vi "PhotoDetSyringeZ.vi"(0 "GoToPhotoDetector":string="G90\nG1 Z0 F100\nG1 X1107.333\tY32.555\nG1\tZ80 F50\nG1\tZ86 F1", 11 "Error In":errorcluster) -> (2 "Vmax":dbl, 3 "Vstart":dbl, 4 "Zfinal":dbl, 10 "VatZfinal":dbl, 13 "Vmin":dbl, 14 "Vmid":dbl, 15 "error out":errorcluster)   [LabVIEW 2019]
panel:
  out "VmidViDiff":dbl[](array[numeric])
  out "ZmidScan":dbl[](array[numeric])
  out "VmidScan":dbl[](array[numeric])
  out "ZstopVminScan":dbl
  out "ZstopVmaxScan":dbl
  out "XYZinLimits":bool
  in  "ZupLim":dbl=89.0 format="%#_7g"
  in  "ZlowLim":dbl=85.0 format="%#_7g"
  in  "YupLim":dbl=32.8 format="%#_7g"
  in  "YlowLim":dbl=32.2 format="%#_7g"
  in  "XupLim":dbl=1107.5 format="%#_7g"
  in  "XlowLim":dbl=1107.0 format="%#_7g"
  in  "Status":string
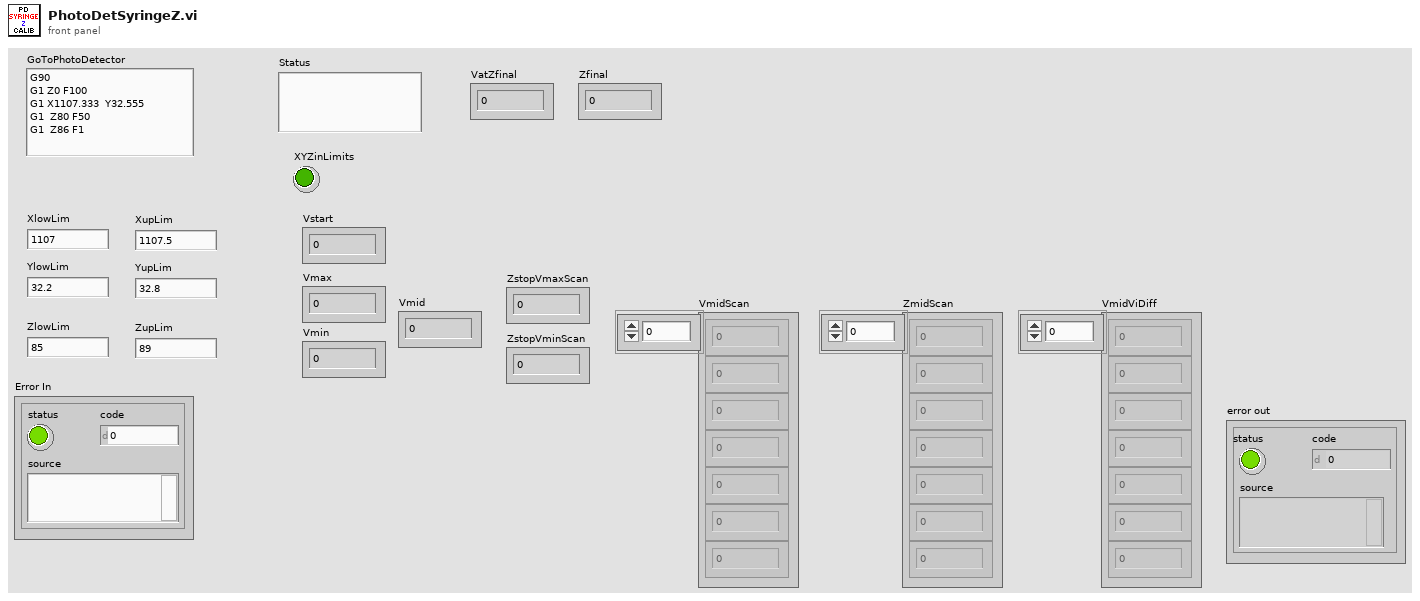
[diagram p1: front panel]
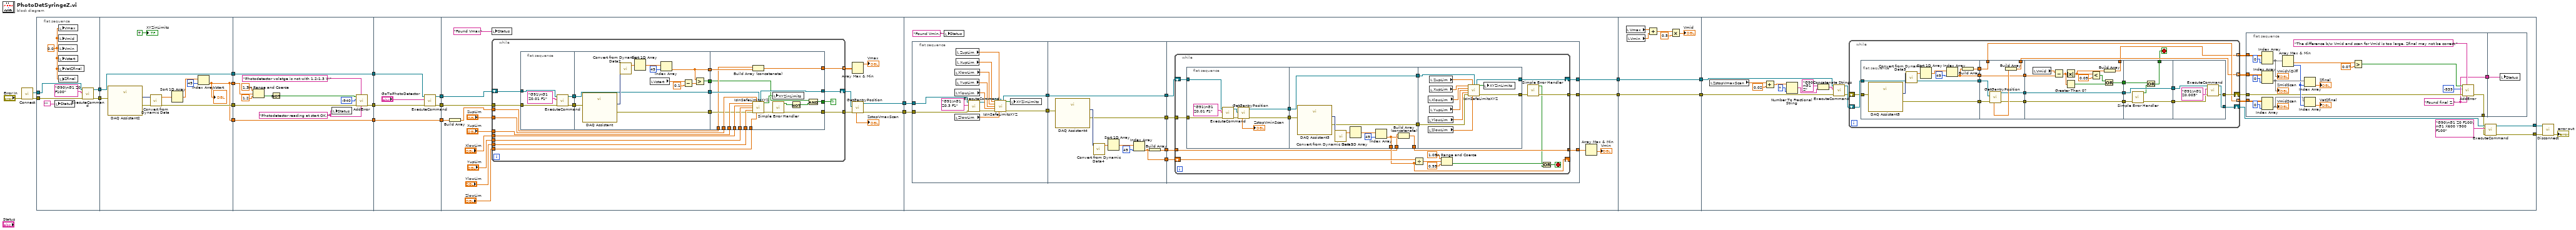
[diagram p0: block diagram]
diagram:
  n1 = call "Connect.vi"("error in (no error)"="Error In") -> ("error out"=w2:errorcluster, "controller"=w1:refnum<k24>)  [unwired: 9 in]
  n2 = flat-sequence {
    tunnel: [w30] -> w24
    tunnel: [w29] -> w19
    tunnel: w2 -> [w27]
    tunnel: w1 -> [w26]
    tunnel: w24 -> [w36]
    tunnel: [w35] -> w23
    tunnel: [w32] -> w22
    tunnel: [w34] -> w20
    tunnel: w19 -> [w34]
    tunnel: [w32] -> w15
    tunnel: w23 -> [w52]
    tunnel: w22 -> [w49]
    tunnel: [w44] -> w21
    tunnel: w20 -> [w44]
    tunnel: [w43] -> w18
    tunnel: w15 -> [w41]
    tunnel: [w41] -> w13
    tunnel: w21 -> [w57]
    tunnel: w18 -> [w56]
    tunnel: [w55] -> w17
    tunnel: [w54] -> w16
    tunnel: [w53] -> w14
    tunnel: w13 -> [w53]
    tunnel: w17 -> [w71]
    tunnel: w16 -> [w76]
    tunnel: w14 -> [w75]
    tunnel: [w61] -> w12
    tunnel: [w60] -> w11
    tunnel: w12 -> [w143]
    tunnel: w11 -> [w144]
    tunnel: [w137] -> w9
    tunnel: [w136] -> w8
    tunnel: w9 -> [w229]
    tunnel: w8 -> [w228]
    tunnel: [w229] -> w7
    tunnel: [w228] -> w6
    tunnel: w7 -> [w247]
    tunnel: w6 -> [w246]
    tunnel: [w231] -> w5
    tunnel: [w234] -> w4
    frame #0 {
      w25 = 0.0 ("Vmax")
      n3 = local write "Status"("") -> ()
      n4 = local write "Vmax"(w25) -> ()
      n5 = local write "Vmid"(w25) -> ()
      n6 = local write "Vmin"(w25) -> ()
      n7 = local write "Vstart"(w25) -> ()
      n8 = local write "VatZfinal"(w25) -> ()
      n9 = local write "Zfinal"(w25) -> ()
      n10 = call "ExecuteCommand.vi"("error in (no error)"=w27, "Command Code"="G90\nG1 Z0 F100", "controller in"=w26) -> ("error out"=w30:errorcluster, "controller out"=w29:refnum<k24>)  [unwired: 6 in, 1 out]
    }
    frame #1 {
      n11 = call "DAQ Assistant2"("error in"=w36) -> ("data"=w40:dynamicdata, "error out"=w35:errorcluster)  [unwired: 16 in, 1 out]
      n12 = call "Convert from Dynamic Data"("Dynamic Data Type"=w40) -> ("Array"=w39:dbl[])  [unwired: 3 in]
      n13 = Sort 1D Array(array=w39) -> (sorted array=w38:dbl[])
      n14 = Index Array(array=w38, index=49) -> (element=w32:dbl)
      "Vstart" <- w32
      "XYZinLimits" <- TRUE ("XYZinLimits")
    }
    frame #2 {
      w42 = "Photodetector reading at start OK." ("NoErrorMessage")
      n15 = In Range and Coerce(upper limit=1.3, x=w49, lower limit=1.2) -> (In Range?=w51:bool)  [unwired: 1 out]
      n16 = Not(x=w51) -> (.not. x?=w47:bool)
      n17 = local write "Status"(w42) -> ()
      n18 = call "AddError.vi"("NoErrorMessage"=w42, "ErrorMessage"="Photodetector volatge is not with 1.2-1.3 V.", "error in"=w52, "code"=-940, "Error?"=w47) -> ("Error out"=w43:errorcluster)  [unwired: 6 in]
    }
    frame #3 {
      n19 = call "ExecuteCommand.vi"("error in (no error)"=w56, "Command Code"="GoToPhotoDetector", "controller in"=w57) -> ("error out"=w55:errorcluster, "controller out"=w54:refnum<k24>)  [unwired: 6 in, 1 out]
    }
    frame #4 {
      n20 = Build Array(w75) -> (w74:dbl[])
      n21 = local write "Status"("Found Vmax" ("NoErrorMessage")) -> ()
      n22 = while {
        shift-right: [w82] -> w64
        shift-left: w76 -> [w95]
        tunnel: "XlowLim" -> [w94]
        tunnel: "XupLim" -> [w93]
        tunnel: "YlowLim" -> [w92]
        tunnel: "YupLim" -> [w91]
        tunnel: "ZupLim" -> [w90]
        tunnel: "ZlowLim" -> [w89]
        tunnel: w74 -> [w83]
        tunnel: [w81] -> w73 mode=indexing
        tunnel: [w80] -> w63
        tunnel: w71 -> [w79]
        stop <- w77 continue-if-true
        n23 = flat-sequence {
          tunnel: w95 -> [w99]
          tunnel: [w98] -> w88
          tunnel: [w97] -> w85
          tunnel: w79 -> [w96]
          tunnel: w88 -> [w108]
          tunnel: [w108] -> w87
          tunnel: [w102] -> w86
          tunnel: w85 -> [w107]
          tunnel: [w104] -> w84
          tunnel: [w101] -> w78
          tunnel: w94 -> [w131]
          tunnel: w93 -> [w130]
          tunnel: w92 -> [w129]
          tunnel: w91 -> [w128]
          tunnel: w90 -> [w127]
          tunnel: w89 -> [w126]
          tunnel: w87 -> [w125]
          tunnel: w86 -> [w123]
          tunnel: w84 -> [w122]
          tunnel: w83 -> [w121]
          tunnel: [w120] -> w82
          tunnel: [w119] -> w81
          tunnel: [w117] -> w80
          tunnel: w78 -> [w116]
          tunnel: [w115] -> w77
          frame #0 {
            n24 = call "ExecuteCommand.vi"("error in (no error)"=w96, "Command Code"="G91\nG1 Z0.01 F1", "controller in"=w99) -> ("error out"=w97:errorcluster, "controller out"=w98:refnum<k24>)  [unwired: 6 in, 1 out]
          }
          frame #1 {
            n25 = call "DAQ Assistant"("error in"=w107) -> ("data"=w112:dynamicdata, "error out"=w102:errorcluster)  [unwired: 16 in, 1 out]
            n26 = call "Convert from Dynamic Data2"("Dynamic Data Type"=w112) -> ("Array"=w111:dbl[])  [unwired: 3 in]
            n27 = Sort 1D Array(array=w111) -> (sorted array=w110:dbl[])
            n28 = local read "Vstart"() -> (w106:dbl)
            n29 = Index Array(array=w110, index=49) -> (element=w104:dbl)
            n30 = Subtract(x=w106, y=0.1) -> (x-y=w103:dbl)
            n31 = Greater?(x=w104, y=w103) -> (0:w101:bool)
          }
          frame #2 {
            n32 = Build Array (concatenate)(w121, w122) -> (w119:dbl[])
            n33 = call "IsInSafeLimitsXYZ.vi"("XupLim"=w130, "ZupLim"=w127, "Controller In"=w125, "XlowLim"=w131, "YupLim"=w128, "YlowLim"=w129, "Error In"=w123, "ZlowLim"=w126) -> ("controller out"=w120:refnum<k24>, "XYZinLimits"=w124:bool, "Error Out"=w118:errorcluster)  [unwired: 5 in]
            n34 = local write "XYZinLimits"(w124) -> ()
            n35 = call <vilib>:"Simple Error Handler.vi"("error in (no error)"=w118) -> ("error?"=w113:bool, "error out"=w117:errorcluster)  [unwired: 4 in, 3 out]
            n36 = Not(x=w113) -> (.not. x?=w114:bool)
            n37 = And(x=w116, y=w114) -> (x .and. y?=w115:bool)
          }
        }
      }
      n38 = Array Max & Min(array=w73) -> (max value=→"Vmax":dbl)  [unwired: 3 out]
      n39 = call "GetGantryPosition.vi"("error in (no error)"=w63, "Controller In"=w64) -> ("error out"=w61:errorcluster, "controller out"=w60:refnum<k24>, "Position Z"=→"ZstopVmaxScan":dbl)  [unwired: 3 in, 4 out]
    }
    frame #5 {
      n40 = flat-sequence {
        tunnel: w144 -> [w158]
        tunnel: w143 -> [w156]
        tunnel: [w146] -> w142
        tunnel: [w147] -> w139
        tunnel: w142 -> [w163]
        tunnel: [w162] -> w141
        tunnel: [w160] -> w140
        tunnel: w139 -> [w161]
        tunnel: [w161] -> w138
        tunnel: [w159] -> w135
        tunnel: w141 -> [w174]
        tunnel: w140 -> [w173]
        tunnel: w138 -> [w172]
        tunnel: [w168] -> w137
        tunnel: [w171] -> w136
        tunnel: w135 -> [w170]
        tunnel: [w169] -> w134
        frame #0 {
          n41 = local read "XlowLim"() -> (w154:dbl)
          n42 = local read "YlowLim"() -> (w152:dbl)
          n43 = local read "ZlowLim"() -> (w150:dbl)
          n44 = local read "ZupLim"() -> (w149:dbl)
          n45 = local read "XupLim"() -> (w153:dbl)
          n46 = local read "YupLim"() -> (w151:dbl)
          n47 = call "ExecuteCommand.vi"("error in (no error)"=w156, "Command Code"="G91\nG1 Z0.3 F1", "controller in"=w158) -> ("error out"=w155:errorcluster, "controller out"=w148:refnum<k24>)  [unwired: 6 in, 1 out]
          n48 = call "IsInSafeLimitsXYZ.vi"("XupLim"=w153, "ZupLim"=w149, "Controller In"=w148, "XlowLim"=w154, "YupLim"=w151, "YlowLim"=w152, "Error In"=w155, "ZlowLim"=w150) -> ("controller out"=w147:refnum<k24>, "XYZinLimits"=w145:bool, "Error Out"=w146:errorcluster)  [unwired: 5 in]
          n49 = local write "XYZinLimits"(w145) -> ()
        }
        frame #1 {
          n50 = call "DAQ Assistant4"("error in"=w163) -> ("data"=w164:dynamicdata, "error out"=w162:errorcluster)  [unwired: 16 in, 1 out]
          n51 = call "Convert from Dynamic Data4"("Dynamic Data Type"=w164) -> ("Array"=w167:dbl[])  [unwired: 3 in]
          n52 = Sort 1D Array(array=w167) -> (sorted array=w166:dbl[])
          n53 = Index Array(array=w166, index=49) -> (element=w160:dbl)
          n54 = Build Array(w160) -> (w159:dbl[])
        }
        frame #2 {
          n55 = while {
            shift-right: [w189] -> _
            shift-left: w173 -> [w190]
            shift-right: [w183] -> w171
            shift-left: w172 -> [w191]
            tunnel: w170 -> [w181]
            tunnel: [w180] -> w169 mode=concatenating
            tunnel: w174 -> [w193]
            tunnel: [w178] -> w168
            stop <- w175 stop-if-true
            n56 = flat-sequence {
              tunnel: w193 -> [w199]
              tunnel: [w195] -> w192
              tunnel: w191 -> [w200]
              tunnel: [w197] -> w185
              tunnel: w192 -> [w207]
              tunnel: [w204] -> w189
              tunnel: w185 -> [w206]
              tunnel: [w206] -> w184
              tunnel: [w205] -> w182
              tunnel: w181 -> [w203]
              tunnel: [w202] -> w180
              tunnel: w184 -> [w215]
              tunnel: [w214] -> w183
              tunnel: w182 -> [w213]
              tunnel: [w212] -> w179
              frame #0 {
                n57 = call "ExecuteCommand.vi"("error in (no error)"=w199, "Command Code"="G91\nG1 Z0.01 F1", "controller in"=w200) -> ("error out"=w194:errorcluster, "controller out"=w198:refnum<k24>)  [unwired: 6 in, 1 out]
                n58 = call "GetGantryPosition.vi"("error in (no error)"=w194, "Controller In"=w198) -> ("error out"=w195:errorcluster, "controller out"=w197:refnum<k24>, "Position Z"=→"ZstopVminScan":dbl)  [unwired: 3 in, 4 out]
              }
              frame #1 {
                n59 = call "DAQ Assistant3"("error in"=w207) -> ("data"=w208:dynamicdata, "error out"=w205:errorcluster)  [unwired: 16 in, 1 out]
                n60 = call "Convert from Dynamic Data3"("Dynamic Data Type"=w208) -> ("Array"=w211:dbl[])  [unwired: 3 in]
                n61 = Sort 1D Array(array=w211) -> (sorted array=w210:dbl[])
                n62 = Index Array(array=w210, index=49) -> (element=w204:dbl)
                n63 = Build Array (concatenate)(w203, w204) -> (w202:dbl[])
              }
              frame #2 {
                n64 = local read "XlowLim"() -> (w222:dbl)
                n65 = local read "YlowLim"() -> (w219:dbl)
                n66 = local read "ZlowLim"() -> (w217:dbl)
                n67 = local read "ZupLim"() -> (w218:dbl)
                n68 = local read "XupLim"() -> (w221:dbl)
                n69 = local read "YupLim"() -> (w220:dbl)
                n70 = call "IsInSafeLimitsXYZ.vi"("XupLim"=w221, "ZupLim"=w218, "Controller In"=w215, "XlowLim"=w222, "YupLim"=w220, "YlowLim"=w219, "Error In"=w213, "ZlowLim"=w217) -> ("controller out"=w214:refnum<k24>, "XYZinLimits"=w216:bool, "Error Out"=w212:errorcluster)  [unwired: 5 in]
                n71 = local write "XYZinLimits"(w216) -> ()
              }
            }
            n72 = Divide(x=w190, y=w189) -> (x/y=w188:dbl)
            n73 = In Range and Coerce(upper limit=1.05, x=w188, lower limit=0.95) -> (In Range?=w177:bool)  [unwired: 1 out]
            n74 = call <vilib>:"Simple Error Handler.vi"("error in (no error)"=w179) -> ("error?"=w176:bool, "error out"=w178:errorcluster)  [unwired: 4 in, 3 out]
            n75 = Or(x=w177, y=w176) -> (x .or. y?=w175:bool)
          }
        }
      }
      n76 = local write "Status"("Found Vmin." ("Status")) -> ()
      n77 = Array Max & Min(array=w134) -> (min value=→"Vmin":dbl)  [unwired: 3 out]
    }
    frame #6 {
      n78 = local read "Vmax"() -> (w226:dbl)
      n79 = local read "Vmin"() -> (w225:dbl)
      n80 = Add(x=w226, y=w225) -> (x+y=w224:dbl)
      n81 = Multiply(x=w224, y=0.5) -> (x*y=→"Vmid":dbl)
    }
    frame #7 {
      n82 = local read "ZstopVmaxScan"() -> (w248:dbl)
      n83 = Add(x=w248, y=0.02) -> (x+y=w249:dbl)
      n84 = Number To Fractional String(number=w249, precision (6)=i16 7) -> (F-format string=w250:string)  [unwired: 2 in]
      n85 = Concatenate Strings("G90\nG1 Z", w250) -> (w242:string)
      n86 = call "ExecuteCommand.vi"("error in (no error)"=w247, "Command Code"=w242, "controller in"=w246) -> ("error out"=w240:errorcluster, "controller out"=w241:refnum<k24>)  [unwired: 6 in, 1 out]
      n87 = while {
        shift-right: [w286] -> w235
        shift-left: w241 -> [w289]
        shift-right: [w283] -> w230
        shift-left: w240 -> [w282]
        tunnel: [w281] -> w237 mode=indexing
        tunnel: [w279] -> w238 mode=indexing
        tunnel: [w272] -> w239 mode=indexing
        stop <- w273 stop-if-true
        n88 = flat-sequence {
          tunnel: w282 -> [w296]
          tunnel: [w295] -> w291
          tunnel: w289 -> [w294]
          tunnel: [w294] -> w288
          tunnel: [w293] -> w285
          tunnel: [w292] -> w280
          tunnel: w291 -> [w307]
          tunnel: [w307] -> w290
          tunnel: w288 -> [w306]
          tunnel: [w305] -> w287
          tunnel: w285 -> [w304]
          tunnel: [w303] -> w284
          tunnel: [w302] -> w281
          tunnel: w280 -> [w302]
          tunnel: [w301] -> w279
          tunnel: w290 -> [w318]
          tunnel: [w313] -> w278
          tunnel: w287 -> [w313]
          tunnel: w284 -> [w310]
          tunnel: [w311] -> w275
          tunnel: [w310] -> w274
          tunnel: [w309] -> w272
          tunnel: w278 -> [w325]
          tunnel: [w325] -> w277
          tunnel: [w320] -> w276
          tunnel: w275 -> [w323]
          tunnel: w274 -> [w322]
          tunnel: [w321] -> w273
          tunnel: w277 -> [w329]
          tunnel: [w328] -> w286
          tunnel: w276 -> [w327]
          tunnel: [w326] -> w283
          frame #0 {
            n89 = call "DAQ Assistant5"("error in"=w296) -> ("data"=w297:dynamicdata, "error out"=w293:errorcluster)  [unwired: 16 in, 1 out]
            n90 = call "Convert from Dynamic Data5"("Dynamic Data Type"=w297) -> ("Array"=w300:dbl[])  [unwired: 3 in]
            n91 = Sort 1D Array(array=w300) -> (sorted array=w299:dbl[])
            n92 = Index Array(array=w299, index=49) -> (element=w295:dbl)
            n93 = Build Array(w295) -> (w292:dbl[])
          }
          frame #1 {
            n94 = call "GetGantryPosition.vi"("error in (no error)"=w304, "Controller In"=w306) -> ("error out"=w303:errorcluster, "controller out"=w305:refnum<k24>, "Position Z"=w308:dbl)  [unwired: 3 in, 4 out]
            n95 = Build Array(w308) -> (w301:dbl[])
          }
          frame #2 {
            n96 = local read "Vmid"() -> (w319:dbl)
            n97 = Subtract(x=w319, y=w318) -> (x-y=w315:dbl)
            n98 = Absolute Value(x=w315) -> (abs(x)=w312:dbl)
            n99 = Greater Than 0?(x=w315) -> (x > 0?=w314:bool)
            n100 = Less?(x=w312, y=0.05) -> (x < y?=w317:bool)
            n101 = Or(x=w317, y=w314) -> (x .or. y?=w311:bool)
            n102 = Build Array(w312) -> (w309:dbl[])
          }
          frame #3 {
            n103 = call <vilib>:"Simple Error Handler.vi"("error in (no error)"=w322) -> ("error?"=w324:bool, "error out"=w320:errorcluster)  [unwired: 4 in, 3 out]
            n104 = Or(x=w323, y=w324) -> (x .or. y?=w321:bool)
          }
          frame #4 {
            n105 = call "ExecuteCommand.vi"("error in (no error)"=w327, "Command Code"="G91\nG1 Z0.005", "controller in"=w329) -> ("error out"=w326:errorcluster, "controller out"=w328:refnum<k24>)  [unwired: 6 in, 1 out]
          }
        }
      }
      n106 = flat-sequence {
        tunnel: w239 -> [w270]
        tunnel: w238 -> [w266]
        tunnel: w237 -> [w265]
        tunnel: w230 -> [w255]
        tunnel: [w254] -> w232
        tunnel: [w252] -> w233
        tunnel: w233 -> [w271]
        frame #0 {
          w252 = "Found final Z." ("Status")
          n107 = Index Array(array=w270, index (col)=0 ("disabled index (col)")) -> (element=w264:dbl[])  [unwired: 1 in]
          "VmidViDiff" <- w264
          n108 = Index Array(array=w266, index (col)=0 ("disabled index (col)")) -> (element=w263:dbl[])  [unwired: 1 in]
          "ZmidScan" <- w263
          n109 = Index Array(array=w265, index (col)=0 ("disabled index (col)")) -> (element=w260:dbl[])  [unwired: 1 in]
          "VmidScan" <- w260
          n110 = Array Max & Min(array=w264) -> (min value=w258:dbl, min index (indices)=w261:i32)  [unwired: 2 out]
          n111 = Index Array(array=w263, index=w261) -> (element=→"Zfinal":dbl)
          n112 = Index Array(array=w260, index=w261) -> (element=→"VatZfinal":dbl)
          n113 = Greater?(x=w258, y=0.07) -> (0:w256:bool)
          n114 = call "AddError.vi"("NoErrorMessage"=w252, "ErrorMessage"="The difference b/w Vmid and scan for Vmid is too large. Zfinal may not be correct.", "error in"=w255, "code"=-939, "Error?"=w256) -> ("Error out"=w254:errorcluster)  [unwired: 6 in]
        }
        frame #1 {
          n115 = local write "Status"(w271) -> ()
        }
      }
      n116 = call "ExecuteCommand.vi"("error in (no error)"=w232, "Command Code"="G90\nG1 Z0 F100\nG1 X600 Y900 F100", "controller in"=w235) -> ("error out"=w231:errorcluster, "controller out"=w234:refnum<k24>)  [unwired: 6 in, 1 out]
    }
  }
  n117 = call "Disconnect.vi"("error in (no error)"=w5, "controller"=w4) -> ("error out"=→"error out":errorcluster)  [unwired: 9 in]
